vi "DB_SelectSum.vi"(8 "error in (no error)":errorcluster, 11 "SQLite Connection in":refnum<class "Connection.lvclass">) -> (0 "error out":errorcluster, 1 "Array - Numeric":dbl[](array[numeric]), 3 "SQLite Connection":refnum<class "Connection.lvclass">)   [LabVIEW 2020]
doc: "Returns how many times each option was chosen using SUM SQL statement."
uses:
  <vilib>/drjdpowell/SQLite Library/SQL Connection/Connection.lvclass
  <vilib>/drjdpowell/SQLite Library/SQL Statement/SQL Statement.lvclass/SQL Statement.ctl
  <vilib>/drjdpowell/SQLite Library/SQL Statement/Column I64.vi
  <vilib>/drjdpowell/SQLite Library/SQL Statement/Error Message.vi
  <vilib>/drjdpowell/SQLite Library/SQL Statement/SQL Statement.lvclass
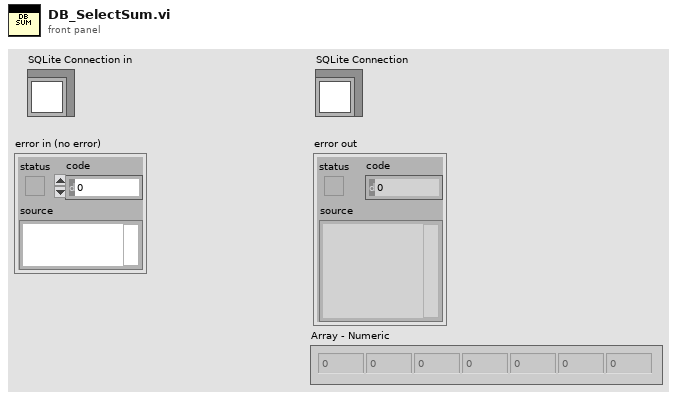
[diagram p1: front panel]
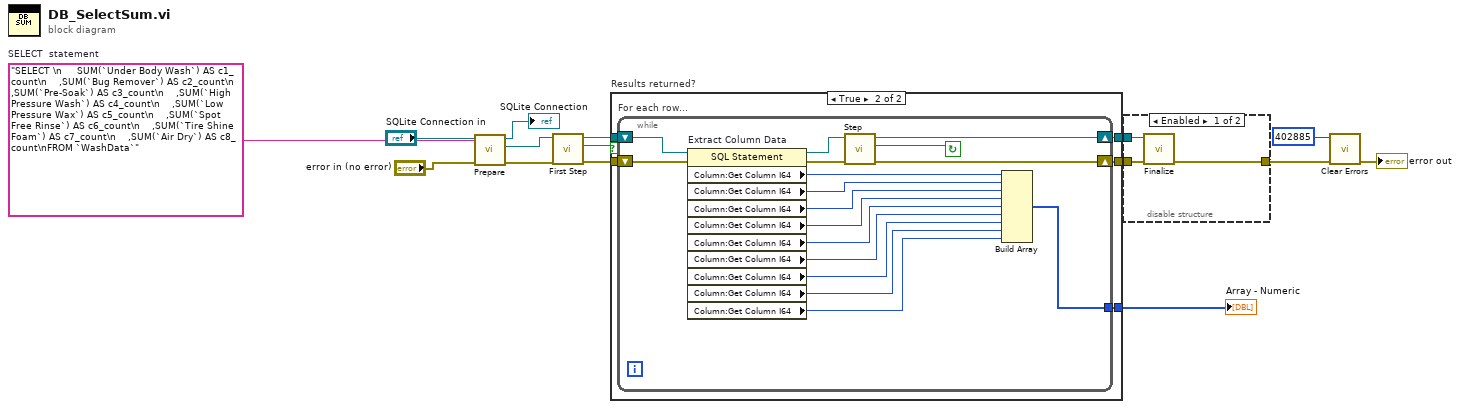
[diagram p0: block diagram]
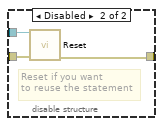
[diagram p2: hidden frame]
diagram:
  w13 = "SELECT \n     SUM(`Under Body Wash`) AS c1_count\n    ,SUM(`Bug Remover`) AS c2_count\n    ,SUM(`Pre-Soak`) AS c3_count\n    ,SUM(`High Pressure Wash`) AS c4_count\n    ,SUM(`Low Pressure Wax`) AS c5_count\n    ,SUM(`Spot Free Rinse`) AS c6_count\n    ,SUM(`Tire Shine Foam`) AS c7_count\n    ,SUM(`Air Dry`) AS c8_count\nFROM `WashData`"  # SELECT  statement
  n1 = call <vilib>:"Prepare.vi"("error in (no error)"="error in (no error)", "SQL"=w13, "SQLite Connection in"="SQLite Connection in") -> ("error out"=w9:errorcluster, "SQL Statement"=w8:refnum<class "SQL Statement.lvclass">, "SQLite Connection"=→"SQLite Connection":refnum<class "Connection.lvclass">)  [unwired: 4 in, 2 out]
  n2 = call <vilib>:"First Step.vi"("error in (no error)"=w9, "SQL Statement in"=w8) -> ("error out"=w11:errorcluster, "Row returned"=w10:bool, "SQL Statement"=w12:refnum<class "SQL Statement.lvclass">)  [unwired: 7 in]
  n3 = case "Results returned?" shown="True" w10 {
    tunnel: [w17 w22] -> w14
    tunnel: [w16 w21] -> w15
    tunnel: w12 -> [w17 w20]
    tunnel: w11 -> [w16 w19]
    tunnel: [_ w18] -> w4
    frame False {
    }
    frame True {
      n4 = while "For each row..." {
        shift-right: [w38] -> w22
        shift-left: w20 -> [w35]
        shift-right: [w36] -> w21
        shift-left: w19 -> [w34]
        tunnel: [w30] -> w18
        stop <- w33 continue-if-true
        n5 = property on="Extract Column Data" class="SQL Statement"(reference=w35, error in=w34) -> (reference out=w39:refnum<class "SQL Statement.lvclass">, error out=w37:errorcluster, "Column:Get Column I64"=w32:i64, "Column:Get Column I64"=w31:i64, "Column:Get Column I64"=w29:i64, "Column:Get Column I64"=w28:i64, "Column:Get Column I64"=w27:i64, "Column:Get Column I64"=w26:i64, "Column:Get Column I64"=w25:i64, "Column:Get Column I64"=w24:i64, "Column:Get Column I64"=w23:i64)
        n6 = call <vilib>:"Step.vi"("error in (no error)"=w37, "SQL Statement in"=w39) -> ("error out"=w36:errorcluster, "Row returned"=w33:bool, "SQL Statement"=w38:refnum<class "SQL Statement.lvclass">)  [unwired: 7 in]
        n7 = Build Array(w32, w31, w29, w28, w27, w26, w25, w24, w23) -> (w30:i64[])
      }
    }
  }
  "Array - Numeric" <- w4
  n8 = disable-structure "Diagram Disable Structure" shown="Enabled" {
    disable-tunnel: w14 -> [w42 w45]
    disable-tunnel: w15 -> [w41 w44]
    disable-tunnel: [w40 w43] -> w2
    frame Enabled {
      n9 = call <vilib>:"Finalize.vi"("error in (no error)"=w41, "SQL Statement in"=w42) -> ("error out"=w40:errorcluster)  [unwired: 9 in]
    }
    frame Disabled {
      # "Reset if you want\nto reuse the statement"
      n10 = call <vilib>:"Reset.vi"("error in (no error)"=w44, "SQL Statement in"=w45) -> ("error out"=w43:errorcluster)  [unwired: 8 in, 1 out]
    }
  }
  n11 = call <vilib>:"Clear Errors.vi"("error in (no error)"=w2, "specific error code to clear (0: all)"=402885) -> ("error out"=→"error out":errorcluster)  [unwired: 4 in, 1 out]
